vi "Get Device Configuration.vi"(8 "error in (no error)":errorcluster, 11 "Device Item Ref in":T2 format="%.0x") -> (0 "error out":errorcluster, 2 "Device Configuration":T1, 3 "Device Item Ref out":T2 format="%.0x")   [LabVIEW 2020, in "NI PXIe-4340 Shared.lvlib"]
uses:
  NI PXIe-4340 Shared.lvlib
  <vilib>/NI VeriStand/Custom Device API/Custom Device Item Ref.ctl
  Device Configuration.ctl
  Constants.vi
  <vilib>/NI VeriStand/Custom Device API/Get Item Property (String).vi
  <vilib>/NI VeriStand/Custom Device API/Get Item Property (Double).vi
  <vilib>/NI VeriStand/Custom Device API/Get Item Property (Variant).vi
  <vilib>/NI VeriStand/Custom Device API/Custom Device API.lvlib
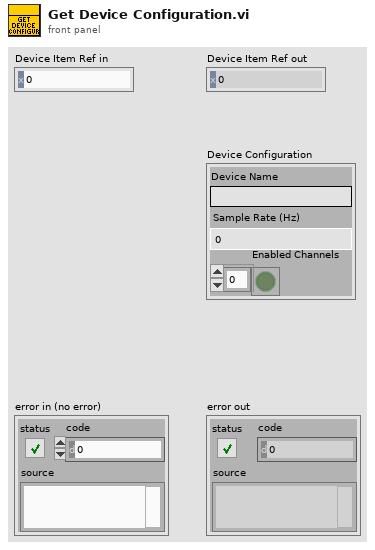
[diagram p1: front panel]
types:
  T1 = typedef "NI PXIe-4340 Shared.lvlib/Device Configuration.ctl" = cluster{"Device Name":string, "Sample Rate (Hz)":dbl, "Enabled Channels":bool[]}
  T2 = typedef "Custom Device API.lvlib/Custom Device Item Ref.ctl" = u64
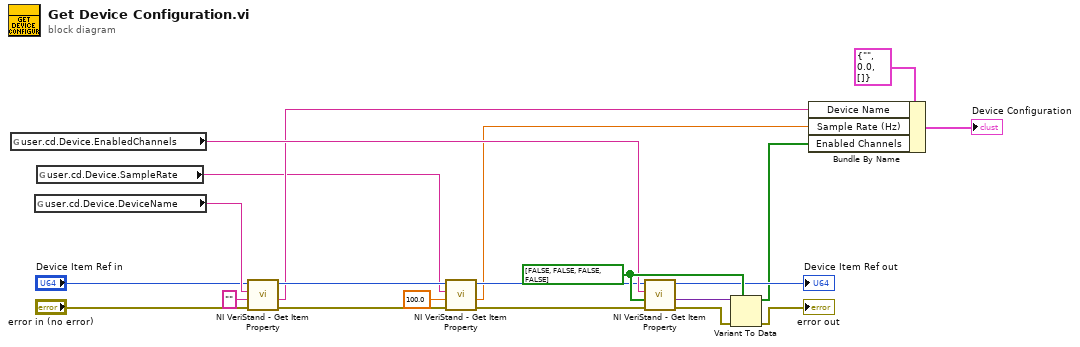
[diagram p0: block diagram]
diagram:
  w21 = bool[] [FALSE, FALSE, FALSE, FALSE]
  n1 = global read "Constants.vi" "user.cd.Device.EnabledChannels"() -> (w15:string)
  n2 = global read "Constants.vi" "user.cd.Device.DeviceName"() -> (w12:string)
  n3 = global read "Constants.vi" "user.cd.Device.SampleRate"() -> (w3:string)
  n4 = call-poly <vilib>:"NI VeriStand - Get Item Property.vi"("error in (no error)"="error in (no error)", "Default Value"="", "Property Name"=w12, "Item Ref in"="Device Item Ref in") -> ("error out"=w5:errorcluster, "Value"=w9:string, "Item Ref out"=w14:T2)  [unwired: 4 in, 1 out]
  n5 = call-poly <vilib>:"NI VeriStand - Get Item Property.vi"("error in (no error)"=w5, "Default Value"=100.0, "Property Name"=w3, "Item Ref in"=w14) -> ("error out"=w4:errorcluster, "Value"=w2:dbl, "Item Ref out"=w6:T2)  [unwired: 4 in, 1 out]
  n6 = call-poly <vilib>:"NI VeriStand - Get Item Property.vi"("error in (no error)"=w4, "Default Value"=w21, "Property Name"=w15, "Item Ref in"=w6) -> ("error out"=w19:errorcluster, "Value"=w17:variant, "Item Ref out"=→"Device Item Ref out":T2)  [unwired: 4 in, 1 out]
  n7 = Variant To Data(error in=w19, type=w21, Variant=w17) -> (data=w7:bool[], error out=→"error out":errorcluster)
  n8 = Bundle By Name(cluster=T1 {"Device Name"="", "Sample Rate (Hz)"=0.0, "Enabled Channels"=[]} ("Device Configuration"), "Device Name"=w9, "Sample Rate (Hz)"=w2, "Enabled Channels"=w7) -> (→"Device Configuration":T1)
